vi "输入电压dc_1.vi"(3 "压电陶瓷电压 (0.1 Vpp)":dbl=0.1, 6 "33522b resource name":refnum<visa-resource-name>) -> ()   [LabVIEW 2019, in "nematic.lvlib"]
uses:
  nematic.lvlib
  lib/Agilent 3352X Series/Agilent 3352X Series.lvlib
panel:
  in  "Channel (1: 1)":i32(ring)=1 items=["1"=1, "2"=2]
  in  "Waveform Function (0: Sine)":i32(ring)=4 items=["Sine"=0, "Square"=1, "Ramp"=2, "Noise"=3, "DC"=4, "Triangle"=5, "Pulse"=6, "Sinc"=11, "D-Lorentz"=12, "Gaussian"=13, "Expo Fall"=14, "Expo Rise"=15, "Haversine"=16]
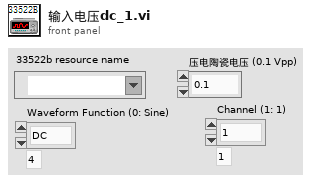
[diagram p1: front panel]
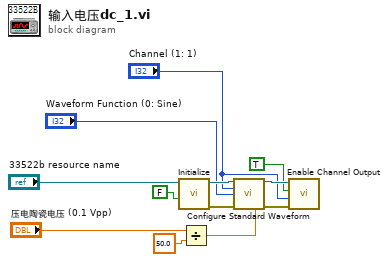
[diagram p0: block diagram]
diagram:
  n1 = call "Initialize.vi"("Reset (Enable)"=FALSE, "VISA resource name"="33522b resource name") -> ("error out"=w9:errorcluster, "VISA resource name out"=w11:refnum<visa-resource-name>)  [unwired: 2 in, 6 out]
  n2 = Divide(x="压电陶瓷电压 (0.1 Vpp)", y=50.0) -> (x/y=w4:dbl)
  n3 = call "Configure Standard Waveform.vi"("VISA resource name"=w11, "Channel (1: 1)"="Channel (1: 1)", "Waveform Function (0: Sine)"="Waveform Function (0: Sine)", "error in (no error)"=w9, "DC Offset (0 V)"=w4) -> ("VISA resource name out"=w10:refnum<visa-resource-name>, "error out"=w8:errorcluster)  [unwired: 5 in, 4 out]
  n4 = call "Enable Channel Output.vi"("error in (no error)"=w8, "Channel (1: 1)"="Channel (1: 1)", "Enable Output (T: Enable)"=TRUE, "VISA resource name"=w10) -> ()  [unwired: 1 in, 7 out]
